vi "Voltage Level Global.vi"() -> ()   [LabVIEW 2018]
panel:
  out "Voltage Level Global":dbl
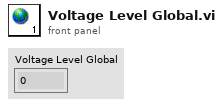
[diagram p1: front panel]
diagram:
